vi "CMN_GetFromEnv.vi"(10 "str in":string) -> (2 "str out":string)   [LabVIEW 2016]
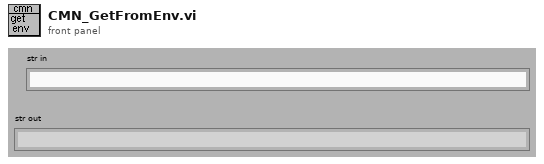
[diagram p1: front panel]
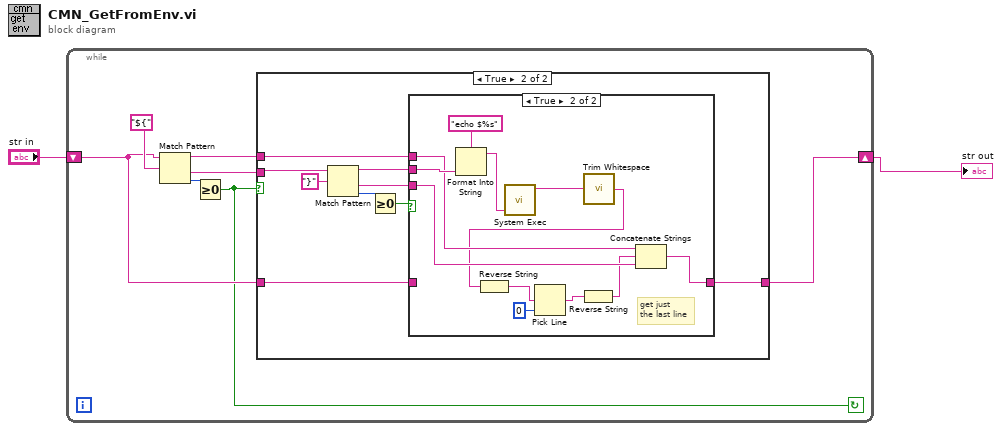
[diagram p0: block diagram]
diagram:
  n1 = while {
    shift-right: [w4] -> w1
    shift-left: "str in" -> [w5]
    stop <- w3 continue-if-true
    n2 = Match Pattern(string=w5, regular expression="${" ("x")) -> (before substring=w6:string, after substring=w7:string, offset past match=w9:i32)  [unwired: 2 out]
    n3 = Greater Or Equal To 0?(x=w9) -> (x >= 0?=w3:bool)
    n4 = case shown="True" w3 {
      tunnel: w5 -> [w10 w15]
      tunnel: [w10 w14] -> w4
      tunnel: w7 -> [_ w19]
      tunnel: w6 -> [_ w12]
      frame False {
      }
      frame True {
        n5 = Match Pattern(string=w19, regular expression="}") -> (before substring=w13:string, after substring=w11:string, offset past match=w17:i32)  [unwired: 2 out]
        n6 = Greater Or Equal To 0?(x=w17) -> (x >= 0?=w16:bool)
        n7 = case shown="True" w16 {
          tunnel: w15 -> [w20 _]
          tunnel: [w20 w26] -> w14
          tunnel: w13 -> [_ w29]
          tunnel: w12 -> [_ w28]
          tunnel: w11 -> [_ w27]
          frame False {
          }
          frame True {
            # "get just \nthe last line"
            n8 = Format Into String(format string="echo $%s", w29) -> (resulting string=w31:string)  [unwired: 2 in, 1 out]
            n9 = call <vilib>:"System Exec.vi"("command line"=w31) -> ("standard output"=w30:string)  [unwired: 5 in, 5 out]
            n10 = call <vilib>:"Trim Whitespace.vi"("string"=w30) -> ("trimmed string"=w25:string)  [unwired: 1 in]
            n11 = Reverse String(1:w25) -> (0:w24:string)
            n12 = Pick Line(multi-line string=w24, line index=0) -> (output string=w22:string)  [unwired: 1 out]
            n13 = Reverse String(1:w22) -> (0:w21:string)
            n14 = Concatenate Strings(w28, w21, w27) -> (w26:string)
          }
        }
      }
    }
  }
  "str out" <- w1
